vi "Deploy Database.vi"() -> ()   [LabVIEW 2014]
panel:
  out "error out":errorcluster
  out "percent complete":u32
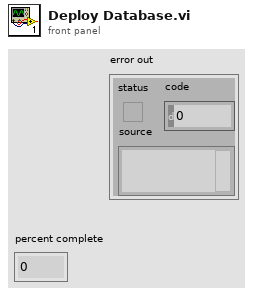
[diagram p1: front panel]
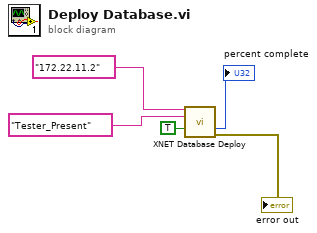
[diagram p0: block diagram]
diagram:
  n1 = call <vilib>:"XNET Database Deploy.vi"("IP address"="172.22.11.2", "alias"="Tester_Present", "wait for complete? (true)"=TRUE) -> ("percent complete"=→"percent complete":u32, "error out"=→"error out":errorcluster)  [unwired: 11 in]
